vi "SpeedM2.vi"(3 "error in (no error)":errorcluster, 4 "Address":u8, 5 "Speed":i32, 6 "VISA Refnum in":refnum<visa-resource-name>) -> (0 "error out":errorcluster, 1 "Valid":bool, 2 "VISA Refnum out":refnum<visa-resource-name>)   [LabVIEW 2015, in "Ion Motion Roboclaw.lvlib"]
uses:
  <instrlib>/Ion Motion Roboclaw/Ion Motion Roboclaw.lvlib
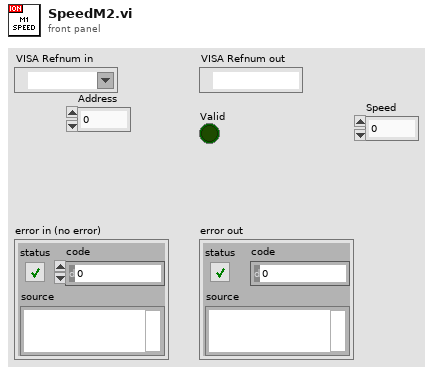
[diagram p1: front panel]
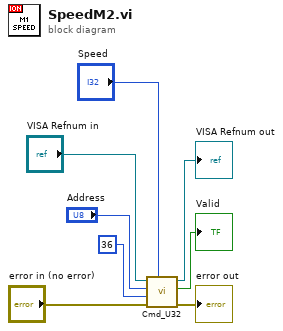
[diagram p0: block diagram]
diagram:
  n1 = call <instrlib>:"Cmd_U32.vi"("Argument"="Speed", "error in (no error)"="error in (no error)", "Cmd"=u8 36, "Address"="Address", "VISA Refnum in"="VISA Refnum in") -> ("error out"=→"error out":errorcluster, "Valid"=→"Valid":bool, "VISA Refnum out"=→"VISA Refnum out":refnum<visa-resource-name>)  [unwired: 4 in]
